vi "ApplyLayoutToObject.vi"(5 "scaling settings":T1={"scaling factor"={"horizontal"=1.0, "vertical"=1.0}, "scale text"=FALSE} {"scaling factor"."vertical" min=0.0; "scaling factor"."horizontal" min=0.0}, 7 "properties to ignore":variant, 8 "error in (no error)":errorcluster, 10 "GObj Refnum":refnum<vi>, 11 "Control Layout in":refnum<class "Control Layout.lvclass">) -> (0 "error out":errorcluster, 3 "Control Layout out":refnum<class "Control Layout.lvclass">)   [LabVIEW 2010, in "NI_SE_Front Panel Layout.lvlib" / "Control Layout.lvclass"]
doc: "Apply layout information to the GObj Refnum."
uses:
  Control Layout.lvclass
  Scaling Factor_Options.ctl
  XY Scaling Factor.ctl
  Object Layout/Object Layout.lvclass
  Control Layout.lvclass/Control Layout.ctl
  Object Layout/Object Layout.lvclass/Object Layout.ctl
  Properties To Ignore.vi
  Set FP Object Size.vi
  NI_SE_Front Panel Layout.lvlib
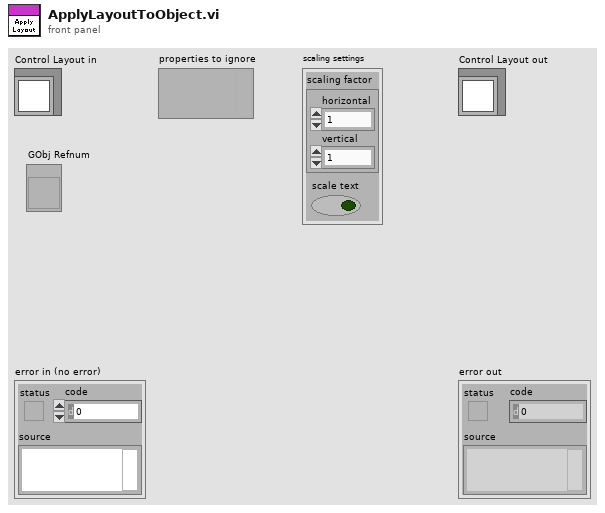
[diagram p1: front panel]
types:
  T1 = typedef "NI_SE_Front Panel Layout.lvlib/Scaling Factor_Options.ctl" = cluster{"scaling factor":T2, "scale text":bool}
  T2 = typedef "NI_SE_Front Panel Layout.lvlib/XY Scaling Factor.ctl" = cluster{"horizontal":dbl, "vertical":dbl}
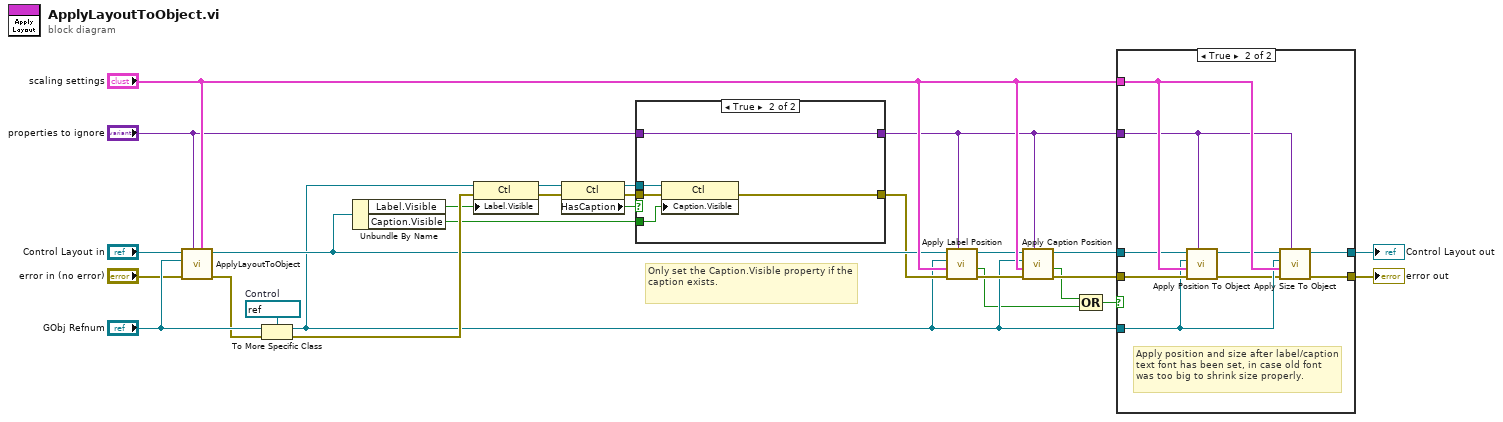
[diagram p0: block diagram]
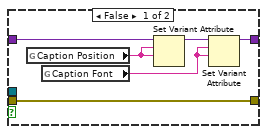
[diagram p3: hidden frame]
diagram:
  w21 = refnum<vi> refnum  # Control
  # "Only set the Caption.Visible property if the caption exists."
  n1 = call-parent "ApplyLayoutToObject.vi"("scaling settings"="scaling settings", "properties to ignore"="properties to ignore", "error in (no error)"="error in (no error)", "GObj Refnum"="GObj Refnum", "Object Layout in"="Control Layout in") -> ("error out"=w25:errorcluster, "Object Layout out"=w9:refnum<class "Control Layout.lvclass">)  [unwired: 5 in]
  n2 = To More Specific Class(target class=w21, reference="GObj Refnum", error in=w25) -> (specific class reference=w3:refnum<vi>, error out=w20:errorcluster)
  n3 = Unbundle By Name(w9) -> ("Label.Visible"=w19:bool, "Caption.Visible"=w14:bool)
  n4 = property class="Ctl"(reference=w3, error in=w20, "Label.Visible"=w19) -> (reference out=w18:refnum<vi>, error out=w17:errorcluster)
  n5 = property class="Ctl"(reference=w18, error in=w17) -> (reference out=w16:refnum<vi>, error out=w15:errorcluster, "HasCaption"=w13:bool)
  n6 = case shown="True" w13 {
    tunnel: w16 -> [_ w39]
    tunnel: w15 -> [w34 w38]
    tunnel: [w34 w37] -> w8
    tunnel: w14 -> [_ w36]
    tunnel: "properties to ignore" -> [w29 w35]
    tunnel: [w30 w35] -> w10
    frame False {
      n7 = global read "Properties To Ignore.vi" "Caption Position"() -> (w32:string)
      n8 = global read "Properties To Ignore.vi" "Caption Font"() -> (w31:string)
      n9 = Set Variant Attribute(Variant=w29, name=w32, value=w32) -> (Variant out=w33:variant)  [unwired: 1 in, 2 out]
      n10 = Set Variant Attribute(Variant=w33, name=w31, value=w31) -> (Variant out=w30:variant)  [unwired: 1 in, 2 out]
    }
    frame True {
      n11 = property class="Ctl"(reference=w39, error in=w38, "Caption.Visible"=w36) -> (error out=w37:errorcluster)  [unwired: 1 out]
    }
  }
  n12 = call "Apply Label Position.vi"("properties to ignore"=w10, "error in (no error)"=w8, "scaling settings"="scaling settings", "Ctl Refnum"=w3, "Control Layout in"=w9) -> ("error out"=w7:errorcluster, "applied?"=w1:bool, "Control Layout out"=w6:refnum<class "Control Layout.lvclass">)  [unwired: 4 in]
  n13 = call "Apply Caption Position.vi"("properties to ignore"=w10, "error in (no error)"=w7, "scaling settings"="scaling settings", "Ctl Refnum"=w3, "Control Layout in"=w6) -> ("error out"=w4:errorcluster, "applied?"=w2:bool, "Control Layout out"=w5:refnum<class "Control Layout.lvclass">)  [unwired: 4 in]
  n14 = Compound Arithmetic op=OR(w2, w1) -> (w12:bool)
  n15 = case shown="True" w12 {
    tunnel: [w40 w50] -> w24
    tunnel: [w41 w49] -> w23
    tunnel: "scaling settings" -> [_ w48]
    tunnel: w10 -> [_ w47]
    tunnel: w5 -> [w40 w46]
    tunnel: w4 -> [w41 w45]
    tunnel: w3 -> [_ w44]
    frame False {
    }
    frame True {
      # "Apply position and size after label/caption text font has been set, in case old font was too big to shrink size properly."
      n16 = call "Apply Position To Object.vi"("properties to ignore"=w47, "error in (no error)"=w45, "scaling settings"=w48, "GObj Refnum"=w44, "NI_SE_Object Layout in"=w46) -> ("error out"=w42:errorcluster, "NI_SE_Object Layout out"=w43:refnum<class "Control Layout.lvclass">)  [unwired: 5 in]
      n17 = call "Apply Size To Object.vi"("properties to ignore"=w47, "error in (no error)"=w42, "scaling settings"=w48, "GObj Refnum"=w44, "NI_SE_Object Layout in"=w43) -> ("error out"=w49:errorcluster, "NI_SE_Object Layout out"=w50:refnum<class "Control Layout.lvclass">)  [unwired: 5 in]
    }
  }
  "error out" <- w23
  "Control Layout out" <- w24
